vi "main.vi"() -> ()   [LabVIEW 2021]
uses:
  MBPOnOff_Controler/typedefs/SetPoint.ctl
  MBPOnOff_Controler/typedefs/Controller_state.ctl
  MBPOnOff_Controler/Model_Predictor/typedefs/Model_v1_parameters.ctl
  <vilib>/OPCUA/controls/NodeId.ctl
  MBPOnOff_Controler/MBPOnOff_Controller.lvlib
  <vilib>/OPCUA/NI OPC UA Client.lvlib
  MBPOnOff_Controler/Model_Predictor/Model_Predictor.lvclass
panel:
  in  "Address to write":string="ns=2;i=2"
  in  "Address to read":string="ns=2;i=3"
  out "AERPUMP":dbl(graph)
  in  "Server endpoint URL":string="opc.tcp://localhost:4840/"
  out "final PWM time":dbl
  in  "Force fixed PWM ON period":bool
  in  "model_v1_parameters":T1={"Sosat"=10.0, "OUR"=0.00175, "R_OUR"=0.0, "T_kLa"=88.0, "R_T_kLa"=0.0, "T0"=27.0, "ku"=0.0006668, "dt"=0.25, "PWM total period"=30.0, "PWM ON period"=2.0, "OUR calc period"=30.0, "OUR calc threshold"=0.01}
  out "PWM2_time":dbl
  out "PWM_control":bool
  out "kLa":dbl
  out "AERPUMP":bool
  out "next state":T2
  in  "Reset":bool
  out "PWM Time":dbl
  out "Oxygen":dbl(graph)
  out "error":bool
  out "CV":bool
  in  "SP":T3={"SPmin"=1.9, "SPmax"=2.1}
  in  "stop":bool
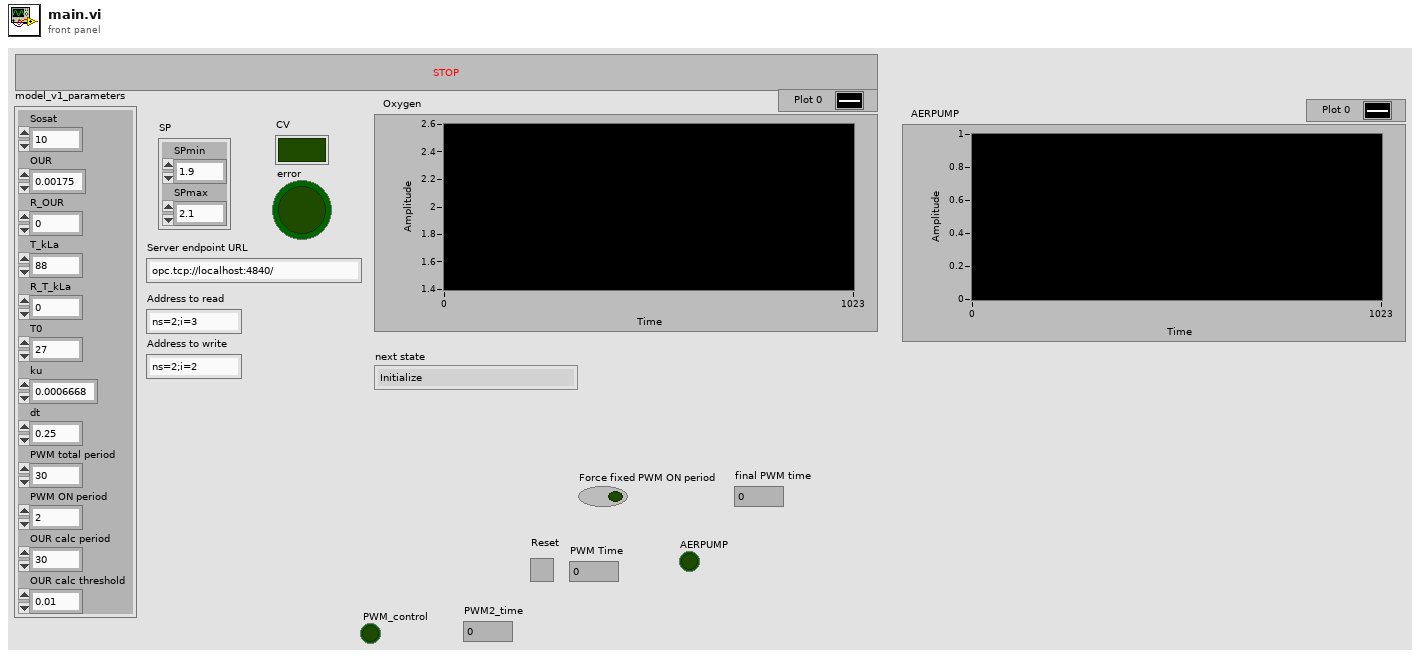
[diagram p1: front panel]
types:
  T1 = typedef "MBPOnOff_Controller.lvlib/Model_Predictor.lvclass/Model_v1_parameters.ctl" = cluster{"Sosat":dbl, "OUR":dbl, "R_OUR":dbl, "T_kLa":dbl, "R_T_kLa":dbl, "T0":dbl, "ku":dbl, "dt":dbl, "PWM total period":dbl, "PWM ON period":dbl, "OUR calc period":dbl, "OUR calc threshold":dbl}
  T2 = typedef "MBPOnOff_Controller.lvlib/Controller_state.ctl" = enum16{"Initialize", "Off_state", "Calculate_Future_Minimum", "On-State", "Calculate_Future_Maximum", "Error"}
  T3 = typedef "MBPOnOff_Controller.lvlib/SetPoint.ctl" = cluster{"SPmin":dbl, "SPmax":dbl}
  T4 = typedef "NodeId.ctl" = string
  T5 = typedef "OPC UA Client Refnum.ctl" = refnum<k21>
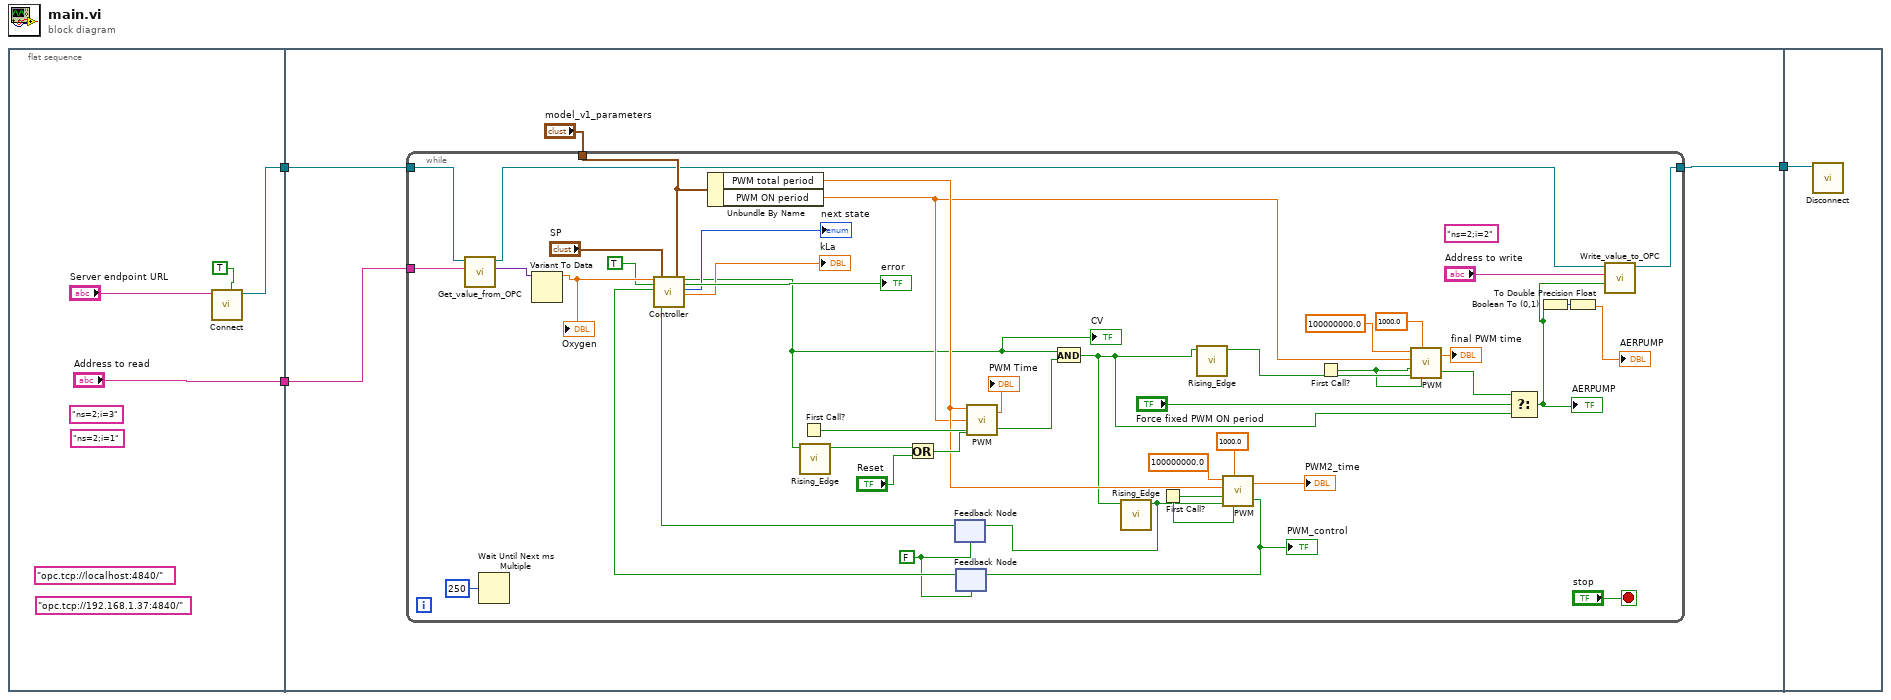
[diagram p0: block diagram]
diagram:
  n1 = flat-sequence {
    tunnel: [w5] -> w3
    tunnel: ["Address to read"] -> w1
    tunnel: w3 -> [w10]
    tunnel: [w9] -> w2
    tunnel: w1 -> [w8]
    tunnel: w2 -> [w56]
    frame #0 {
      (unwired) T4 "ns=2;i=1" ("node ID")
      (unwired) T4 "ns=2;i=3" ("node ID")
      (unwired) "opc.tcp://192.168.1.37:4840/" ("server endpoint URL")
      (unwired) "opc.tcp://localhost:4840/" ("server endpoint URL")
      n2 = call <vilib>:"Connect.vi"("trust any server (F)"=TRUE, "server endpoint URL"="Server endpoint URL") -> ("OPC UA client refnum out"=w5:T5)  [unwired: 7 in, 2 out]
    }
    frame #1 {
      n3 = while {
        tunnel: "model_v1_parameters" -> [w36]
        tunnel: w10 -> [w23]
        tunnel: [w12] -> w9
        tunnel: w8 -> [w18]
        stop <- "stop" stop-if-true
        (unwired) T4 "ns=2;i=2" ("node ID")
        w33 = FALSE
        n4 = call "Get_value_from_OPC.vi"("Address to read"=w18, "OPC UA client refnum in"=w23) -> ("Data out"=w22:variant, "OPC UA client refnum out"=w13:T5)  [unwired: 5 in, 1 out]
        n5 = Wait Until Next ms Multiple(millisecond multiple=u32 250) -> ()  [unwired: 1 out]
        n6 = Variant To Data(Variant=w22) -> (data=w21:dbl)  [unwired: 2 in, 1 out]
        "Oxygen" <- w21
        n7 = Unbundle By Name(w36) -> ("PWM total period"=w37:dbl, "PWM ON period"=w27:dbl)
        n8 = First Call?() -> (First Call?: T/F=w52:bool)
        n9 = feedback #1(w33) -> (w34:bool)
        n10 = feedback #2(w33) -> (w42:bool)
        n11 = call "Controller.vi"("y"=w21, "Enable_Predicting_control"=TRUE, "CV"=w42, "SP"="SP", "real pwm rising edge"=w34, "model_v1_parameters"=w36) -> ("CV"=w15:bool, "error"=→"error":bool, "next state"=→"next state":T2, "kLa out"=→"kLa":dbl)  [unwired: 10 in]
        "CV" <- w15
        n12 = call "Rising_Edge.vi"("input"=w15) -> ("rising_edge"=w47:bool)  [unwired: 10 in]
        n13 = Or(x=w47, y="Reset") -> (x .or. y?=w48:bool)
        n14 = call "PWM.vi"("Reset"=w48, "Initialize?"=w52, "On Period"=w27, "Total Period"=w37) -> ("OUTPUT"=w43:bool, "Time"=→"PWM Time":dbl)  [unwired: 2 in]
        n15 = And(x=w15, y=w43) -> (x .and. y?=w31:bool)
        n16 = call "Rising_Edge.vi"("input"=w31) -> ("rising_edge"=w35:bool)  [unwired: 10 in]
        n17 = feedback-in #1(w35) -> ()
        n18 = First Call?() -> (First Call?: T/F=w38:bool)
        n19 = call "Rising_Edge.vi"("input"=w31) -> ("rising_edge"=w28:bool)  [unwired: 10 in]
        n20 = call "PWM.vi"("Force time?"=w38, "Forced Time"=1000.0, "Reset"=w35, "Initialize?"=w38, "On Period"=w37, "Total Period"=100000000.0) -> ("OUTPUT"=w41:bool, "Time"=→"PWM2_time":dbl)
        "PWM_control" <- w41
        n21 = feedback-in #2(w41) -> ()
        n22 = First Call?() -> (First Call?: T/F=w26:bool)
        n23 = call "PWM.vi"("Force time?"=w26, "Forced Time"=1000.0, "Reset"=w28, "Initialize?"=w26, "On Period"=w27, "Total Period"=100000000.0) -> ("OUTPUT"=w25:bool, "Time"=→"final PWM time":dbl)
        n24 = Select(t=w25, s="Force fixed PWM ON period", f=w31) -> (s? t:f=w16:bool)
        "AERPUMP" <- w16
        n25 = Boolean To (0,1)(Boolean=w16) -> (0, 1=w20:i16)
        n26 = To Double Precision Float(number=w20) -> (double precision float=→"AERPUMP":dbl)
        n27 = call "Write_value_to_OPC.vi"("Data in"=w16, "Address to write"="Address to write", "OPC UA client refnum in"=w13) -> ("OPC UA client refnum out"=w12:T5)  [unwired: 8 in]
      }
    }
    frame #2 {
      n28 = call <vilib>:"Disconnect.vi"("OPC UA client refnum in"=w56) -> ()  [unwired: 10 in, 1 out]
    }
  }
